vi "Advanced SCP File Upload.vi"() -> ()   [LabVIEW 2018]
doc: "Uploads, or sends, any local file to a remote SSH server in an efficient, iterative manner. This is similar to the SCP command line utility when transferring, or copying, a local file to a remote destination. Provides advanced functionality for measuring and monitoring transfer performance."
uses:
  Toolkit/Type Definitions/Permissions.ctl
  Toolkit/Type Definitions/Modes.ctl
  Toolkit/Session/Support/Create from SSH.vi
  Toolkit/Session/Support/Password Authentication.vi
  Toolkit/Channel/Support/Create from SCP Send.vi
  Toolkit/Channel/Support/Destroy to Session.vi
  Toolkit/Session/Support/Destroy to SSH.vi
  Toolkit/SSH/SSH.lvclass
  Toolkit/Session/Session.lvclass
  Toolkit/Channel/Channel.lvclass
  Toolkit/Toolkit.lvlib
panel:
  out "File Upload Time":dbl format="%<%H:%M:%S%3u>t"
  out "File Upload Rate":dbl format="%.3p"
  out "Block Upload Rate":dbl format="%.3p"
  out "Bytes Uploaded":u64
  in  "Abort Upload":bool
  out "Upload Progress":dbl(slide) scale=0.0..1.0
  in  "Block Size":i32=30000 min=0 max=30000
  in  "Remote File":string
  in  "Local File":path
  in  "Remote SSH Server":string
  in  "Password":string
  in  "Username":string
  # "Overview: Demonstrates transferring, or uploading, a local file to a remote SSH server, similar to the SCP command line utility, with advanced functionality\nInstructions:\n1. Enter the IP address or host name of the remote SSH server. This can be a CompactRIO (cRIO) running the National Instruments Linux Real-Time (NI Linux RT) operating system with the Enable Secure Shell Server (sshd) checkbox checked. \n2. Enter a username. If using a cRIO with a default configuration, then the username is \"admin\".\n3. Enter a password for the username. If using a cRIO with a default configuration, then the password is blank (empty).\n4. Select a file on the local computer to transfer/upload to the remote SSH server.\n5. Enter a path and/or filename for the uploaded file on the remote SSH server. Typically, this is a POSIX/UNIX file path with a backslash, \"/\", use to separate directories and the default directory is the remote user's home directory, i.e. \"/home/admin\" on a default configured cRIO.\n6. Run this VI."
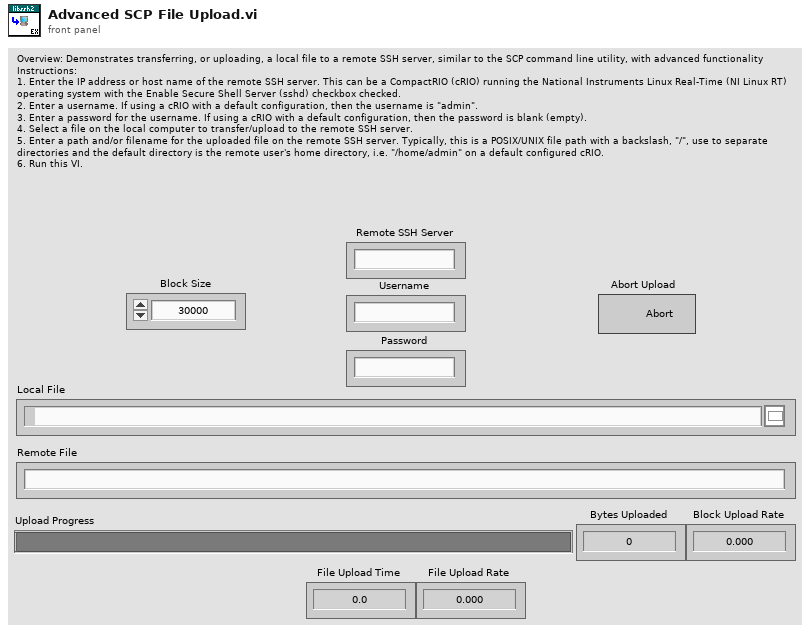
[diagram p1: front panel]
types:
  T1 = enum16{"open", "replace", "create", "open or create", "replace or create", "replace or create with confirmation"}
  T2 = typedef "Toolkit.lvlib/Permissions.ctl" = cluster{"Owner":T3, "Group":T3, "Others":T3}
  T3 = typedef "Toolkit.lvlib/Modes.ctl" = cluster{"Read":bool, "Write":bool, "Execute":bool}
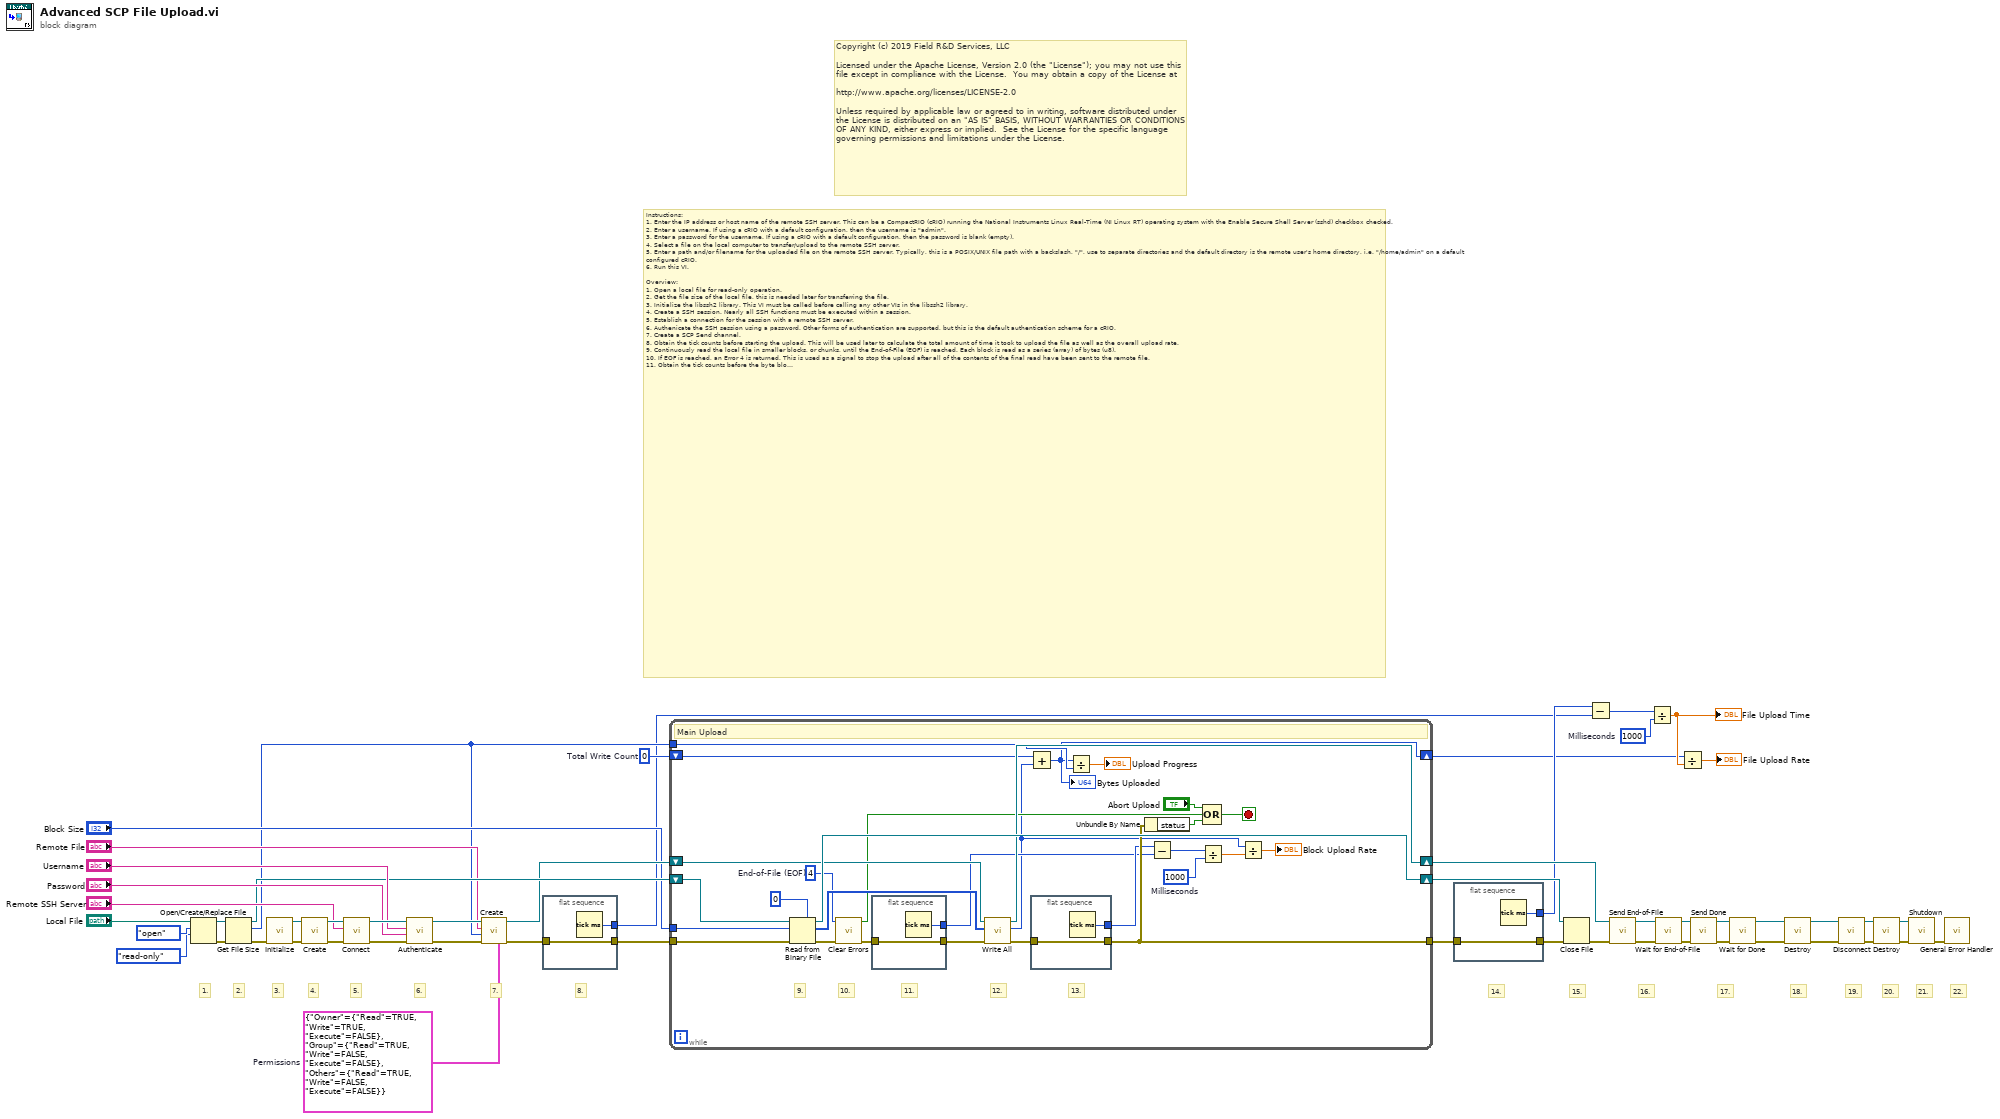
[diagram p0: block diagram]
diagram:
  w4 = u32 1000  # Milliseconds
  w13 = u64 0  # Total Write Count
  w40 = T2 {"Owner"={"Read"=TRUE, "Write"=TRUE, "Execute"=FALSE}, "Group"={"Read"=TRUE, "Write"=FALSE, "Execute"=FALSE}, "Others"={"Read"=TRUE, "Write"=FALSE, "Execute"=FALSE}}  # Permissions
  # "Copyright (c) 2019 Field R&D Services, LLC\n\nLicensed under the Apache License, Version 2.0 (the \"License\"); you may not use this file except in compliance with the License.  You may obtain a copy of the License at\n\nhttp://www.apache.org/licenses/LICENSE-2.0\n\nUnless required by applicable law or agreed to in writing, software distributed under the License is distributed on an \"AS IS\" BASIS, WITHOUT WARRANTIES OR CONDITIONS OF ANY KIND, either express or implied.  See the License for the specific language governing permissions and limitations under the License."
  # "22."
  # "21."
  # "20."
  # "19."
  # "18."
  # "17."
  # "16."
  # "15."
  # "14."
  # "8."
  # "7."
  # "6."
  # "5."
  # "4."
  # "3."
  # "2."
  # "1."
  # "Instructions:\n1. Enter the IP address or host name of the remote SSH server. This can be a CompactRIO (cRIO) running the National Instruments Linux Real-Time (NI Linux RT) operating system with the Enable Secure Shell Server (sshd) checkbox checked. \n2. Enter a username. If using a cRIO with a default configuration, then the username is \"admin\".\n3. Enter a password for the username. If using a cRIO with a default configuration, then the password is blank (empty).\n4. Select a file on the local computer to transfer/upload to the remote SSH server.\n5. Enter a path and/or filename for the uploaded file on the remote SSH server. Typically, this is a POSIX/UNIX file path with a backslash, \"/\", use to separate directories and the default directory is the remote user's home directory, i.e. \"/home/admin\" on a default configured cRIO.\n6. Run this VI.\n\nOverview:\n1. Open a local file for read-only operation.\n2. Get the file size of the local file, this is needed later for transferring the file.\n3. Initialize the libssh2 library. This VI must be called before calling any other VIs in the libssh2 library.\n4. Create a SSH session. Nearly all SSH functions must be executed within a session.\n5. Establish a connection for the session with a remote SSH server.\n6. Authenicate the SSH session using a password. Other forms of authentication are supported, but this is the default authentication scheme for a cRIO. \n7. Create a SCP Send channel.\n8. Obtain the tick counts before starting the upload. This will be used later to calculate the total amount of time it took to upload the file as well as the overall upload rate.\n9. Continuously read the local file in smaller blocks, or chunks, until the End-of-File (EOF) is reached. Each block is read as a series (array) of bytes (u8).\n10. If EOF is reached, an Error 4 is returned. This is used as a signal to stop the upload after all of the contents of the final read have been sent to the remote file.\n11. Obtain the tick counts before the byte block from the local file is sent to the remote file. This will be used to calculate the upload, or transfer, rate of the block.\n12. Write all of the bytes from the block, or chunk, not the entire file. Note, this will silently overwrite any existing file on the remote SSH server with the same path and file name.\n13. Obtain the tick counts after the block, or chunk, has been sent to the remote file. This is used to calculate the block upload rate.\n14. Obtain the tick counts after the entire file has been uploaded to the remote SSH server. THis is used to calculate the file upload rate and total amount of time to upload the entire file.\n15. Close the local file resource. This is not strictly necessary, but it is good practice.\n16. Tell the remote SSH server that all of the bytes from the local file have been sent to it and no more bytes will be sent. Also, wait for the remote SSH server to acknowledge that the file transfer is complete. This is not strictly required, but it is good practice.\n17. Close the SCP Send channel. Again, not strictly required, but it is good practice.\n18. Destroy the SCP Send channel. Since the \"Create\" VI is used, the complementary \"Destroy\" VI must be used to free resources within the libssh2 library.\n19. Disconnect from the remote SSH server.\n20. Destroy the session to free resources within the libssh2 library.\n21. Shutdown the libssh2 library. This VI must be last VI called for the libssh2 library. No other libssh2 VIs should be called once this VI is executed.\n22. Provide some error handling and reporting. Libssh2 errors will be in the -8100 range."
  n1 = Open/Create/Replace File(file path (use dialog)="Local File", operation (0:open)=T1."open", access (0:read/write)=enum16{"read/write", "read-only", "write-only"}."read-only") -> (refnum out=w41:refnum<file>, error out=w42:errorcluster)  [unwired: 3 in, 1 out]
  n2 = Get File Size(file=w41, error in=w42) -> (refnum out=w39:refnum<file>, size (in bytes)=w12:i64, 0:w15:errorcluster)
  n3 = call "Initialize.vi"("Error In"=w15) -> ("Error Out"=w52:errorcluster, "SSH"=w53:refnum<class "SSH.lvclass">)  [unwired: 9 in]
  n4 = call-poly "Create.vi"("Error In"=w52, "SSH"=w53) -> ("Error Out"=w50:errorcluster, "Sesssion"=w51:refnum<class "Session.lvclass">)  [unwired: 8 in]
  n5 = call "Connect.vi"("Error In"=w50, "Address"="Remote SSH Server", "Session In"=w51) -> ("Error Out"=w48:errorcluster, "Sesssion Out"=w49:refnum<class "Session.lvclass">)  [unwired: 7 in]
  n6 = call-poly "Authenticate.vi"("Error In"=w48, "Password"="Password", "Username"="Username", "Session In"=w49) -> ("Error Out"=w43:errorcluster, "Sesssion Out"=w44:refnum<class "Session.lvclass">)  [unwired: 6 in]
  n7 = call-poly "Create.vi"("Permissions"=w40, "Error In"=w43, "File Size"=w12, "Remote Destination Path"="Remote File", "Session"=w44) -> ("Error Out"=w11:errorcluster, "Channel"=w18:refnum<class "Channel.lvclass">)  [unwired: 5 in]
  n8 = flat-sequence {
    tunnel: w11 -> [w55]
    tunnel: [w55] -> w10
    tunnel: [w54] -> w6
    frame #0 {
      n9 = Tick Count (ms)() -> (millisecond timer value=w54:u32)
    }
  }
  n10 = while {
    shift-right: [w82] -> w38
    shift-left: w39 -> [w84]
    shift-right: [w77] -> w17
    shift-left: w18 -> [w76]
    tunnel: w10 -> [w81]
    tunnel: "Block Size" -> [w80]
    shift-right: [w56] -> w2
    shift-left: w13 -> [w75]
    tunnel: w12 -> [w73]
    tunnel: [w66] -> w9
    stop <- w64 stop-if-true
    w60 = u32 1000  # Milliseconds
    w74 = 4  # End-of-File (EOF)
    # "13."
    # "12."
    # "11."
    # "10."
    # "9."
    # "Main Upload"
    n11 = Read from Binary File(5:u8 0, 8:w81, 10:w80, 11:w84) -> (0:w79:errorcluster, 2:w78:u8[], 3:w82:refnum<file>)  [unwired: 2 in, 1 out]
    n12 = call <vilib>:"Clear Errors.vi"("error in (no error)"=w79, "specific error code to clear (0: all)"=w74) -> ("error out"=w71:errorcluster, "specific error cleared?"=w67:bool)  [unwired: 4 in]
    n13 = flat-sequence {
      tunnel: w71 -> [w88]
      tunnel: [w88] -> w70
      tunnel: [w87] -> w62
      frame #0 {
        n14 = Tick Count (ms)() -> (millisecond timer value=w87:u32)
      }
    }
    n15 = call "Write All.vi"("Error In"=w70, "Data"=w78, "Channel In"=w76) -> ("Error Out"=w69:errorcluster, "Write Count"=w57:u64, "Channel Out"=w77:refnum<class "Channel.lvclass">)  [unwired: 5 in, 1 out]
    n16 = Add(x=w75, y=w57) -> (x+y=w56:u64)
    "Bytes Uploaded" <- w56
    n17 = flat-sequence {
      tunnel: w69 -> [w86]
      tunnel: [w86] -> w66
      tunnel: [w85] -> w63
      frame #0 {
        n18 = Tick Count (ms)() -> (millisecond timer value=w85:u32)
      }
    }
    n19 = Divide(x=w56, y=w73) -> (x/y=→"Upload Progress":dbl)
    n20 = Unbundle By Name(w66) -> ("status"=w65:bool)
    n21 = Subtract(x=w63, y=w62) -> (x-y=w61:u32)
    n22 = Divide(x=w61, y=w60) -> (x/y=w59:dbl)
    n23 = Compound Arithmetic op=OR("Abort Upload", w67, w65) -> (w64:bool)
    n24 = Divide(x=w57, y=w59) -> (x/y=→"Block Upload Rate":dbl)
  }
  n25 = flat-sequence {
    tunnel: w9 -> [w90]
    tunnel: [w90] -> w8
    tunnel: [w89] -> w7
    frame #0 {
      n26 = Tick Count (ms)() -> (millisecond timer value=w89:u32)
    }
  }
  n27 = Close File(refnum=w38, error in=w8) -> (error out=w16:errorcluster)  [unwired: 1 out]
  n28 = Subtract(x=w7, y=w6) -> (x-y=w5:u32)
  n29 = call "Send End-of-File.vi"("Error In"=w16, "Channel In"=w17) -> ("Error Out"=w36:errorcluster, "Channel Out"=w37:refnum<class "Channel.lvclass">)  [unwired: 8 in]
  n30 = Divide(x=w5, y=w4) -> (x/y=w3:dbl)
  "File Upload Time" <- w3
  n31 = call "Wait for End-of-File.vi"("Error In"=w36, "Channel In"=w37) -> ("Error Out"=w27:errorcluster, "Channel Out"=w28:refnum<class "Channel.lvclass">)  [unwired: 8 in]
  n32 = Divide(x=w2, y=w3) -> (x/y=→"File Upload Rate":dbl)
  n33 = call "Send Done.vi"("Error In"=w27, "Channel In"=w28) -> ("Error Out"=w25:errorcluster, "Channel Out"=w26:refnum<class "Channel.lvclass">)  [unwired: 8 in]
  n34 = call "Wait for Done.vi"("Error In"=w25, "Channel In"=w26) -> ("Error Out"=w23:errorcluster, "Channel Out"=w24:refnum<class "Channel.lvclass">)  [unwired: 8 in]
  n35 = call-poly "Destroy.vi"("Error In"=w23, "Channel"=w24) -> ("Error Out"=w34:errorcluster, "Session"=w35:refnum<class "Session.lvclass">)  [unwired: 8 in]
  n36 = call "Disconnect.vi"("Error In"=w34, "Session In"=w35) -> ("Error Out"=w32:errorcluster, "Sesssion Out"=w33:refnum<class "Session.lvclass">)  [unwired: 8 in]
  n37 = call-poly "Destroy.vi"("Error In"=w32, "Session"=w33) -> ("Error Out"=w30:errorcluster, "SSH"=w31:refnum<class "SSH.lvclass">)  [unwired: 8 in]
  n38 = call "Shutdown.vi"("Error In"=w30, "SSH"=w31) -> ("Error Out"=w29:errorcluster)  [unwired: 9 in]
  n39 = call <vilib>:"General Error Handler.vi"("error in (no error)"=w29) -> ()  [unwired: 10 in, 5 out]
